vi "Retrieve_GetImage.vi"(6 "File and Directory Blacklist":string[](array[string]), 8 "error in (no error)":errorcluster, 9 "Image Metadata in":T2={"title"="", "description"="", "ID"="", "version"="", "component type"=5} {"component type" items=["standard", "hidden", "system", "unknown", "startup", "image", "essential"]}, 10 "Image Filepath":path, 11 "DevInfo":T1={"Hostname"="", "IPAddress"="", "MAC"="", "SerialNum"="", "Model"="", "Status"="", "FW"="", "OSDesc"="", "ImgTitle"="", "ImgDesc"="", "ImgVer"="", "ImgID"="", "IP Address Request Mode"=1, "SubnetMask"="", "Gateway"="", "DNSServer"=""} {"IP Address Request Mode" items=["Static"=1, "DHCP/Link-Local"=2, "Link-Local Only"=4, "DHCP Only"=8]}) -> (0 "error out":errorcluster)   [LabVIEW 2021]
uses:
  <vilib>/nisyscfg/Software 1.2.ctl
  <vilib>/nisyscfg/Component Type.ctl
  TypeDefs/DevInfo.ctl
  TypeDefs/TargetAccess.ctl
  <vilib>/nisyscfg/Create System Image (File).vi
  <vilib>/nisyscfg/Close (System).vi
  <vilib>/nisyscfg/nisyscfg.lvlib
panel:
  out "Progress":i8(slide) scale=0.0..100.0
  out "Status":string
  in  "Stop Checking for Events":bool
  # "Retrieving application image..."
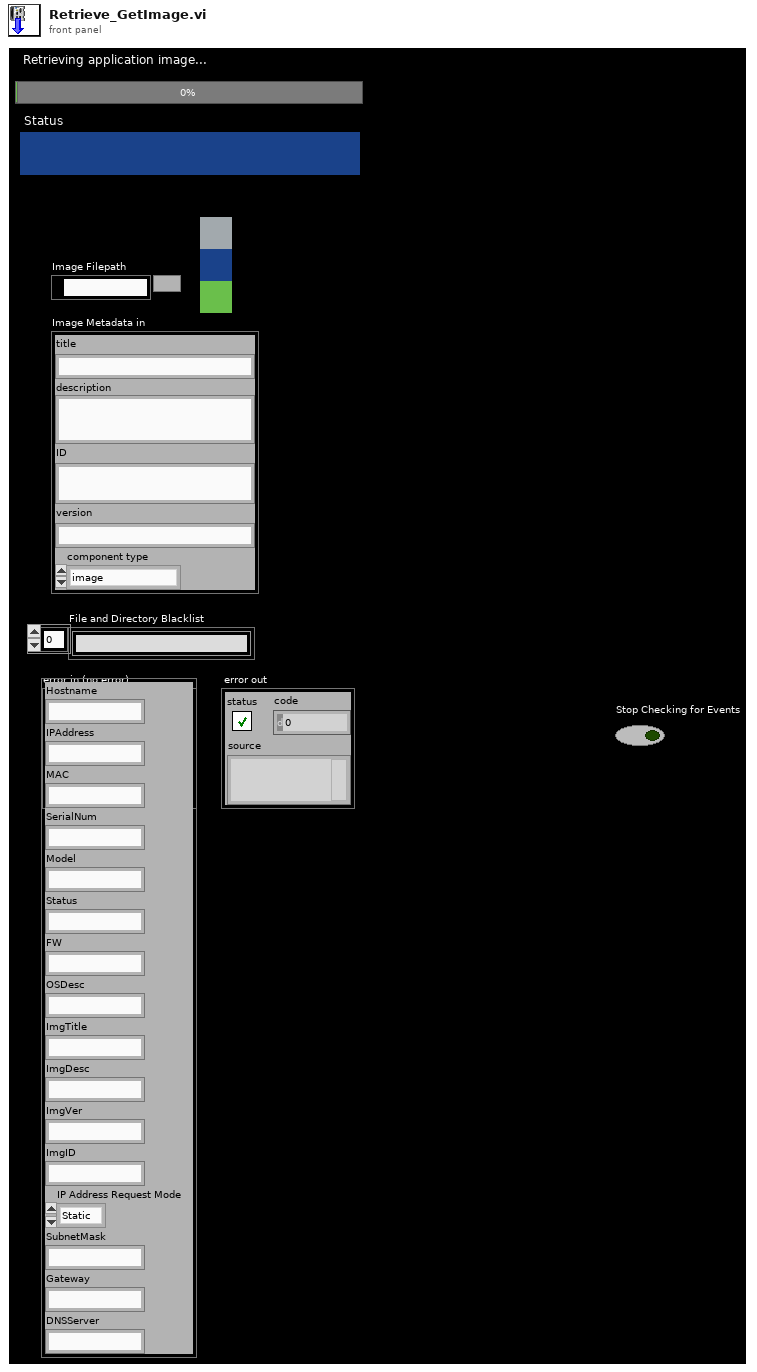
[diagram p1: front panel]
types:
  T1 = typedef "DevInfo.ctl" = cluster{"Hostname":string, "IPAddress":string, "MAC":string, "SerialNum":string, "Model":string, "Status":string, "FW":string, "OSDesc":string, "ImgTitle":string, "ImgDesc":string, "ImgVer":string, "ImgID":string, "IP Address Request Mode":i32, "SubnetMask":string, "Gateway":string, "DNSServer":string}
  T2 = typedef "nisyscfg.lvlib/Software 1.2.ctl" = cluster{"title":string, "description":string, "ID":string, "version":string, "component type":T3}
  T3 = typedef "nisyscfg.lvlib/Component Type.ctl" = u32
  T4 = typedef "TargetAccess.ctl" = enum16{"Read-Only", "Admin"}
  T5 = enum32{"state changed", "beginning restart", "getting file", "putting file", "creating directory", "deleting file", "deleting directory", "enumerating file system", "renaming file", "current component", "operation progress", "downloading file", "unpacking file", "running install script", "creating image", "validating image", "applying image", "beginning format", "completing format"}
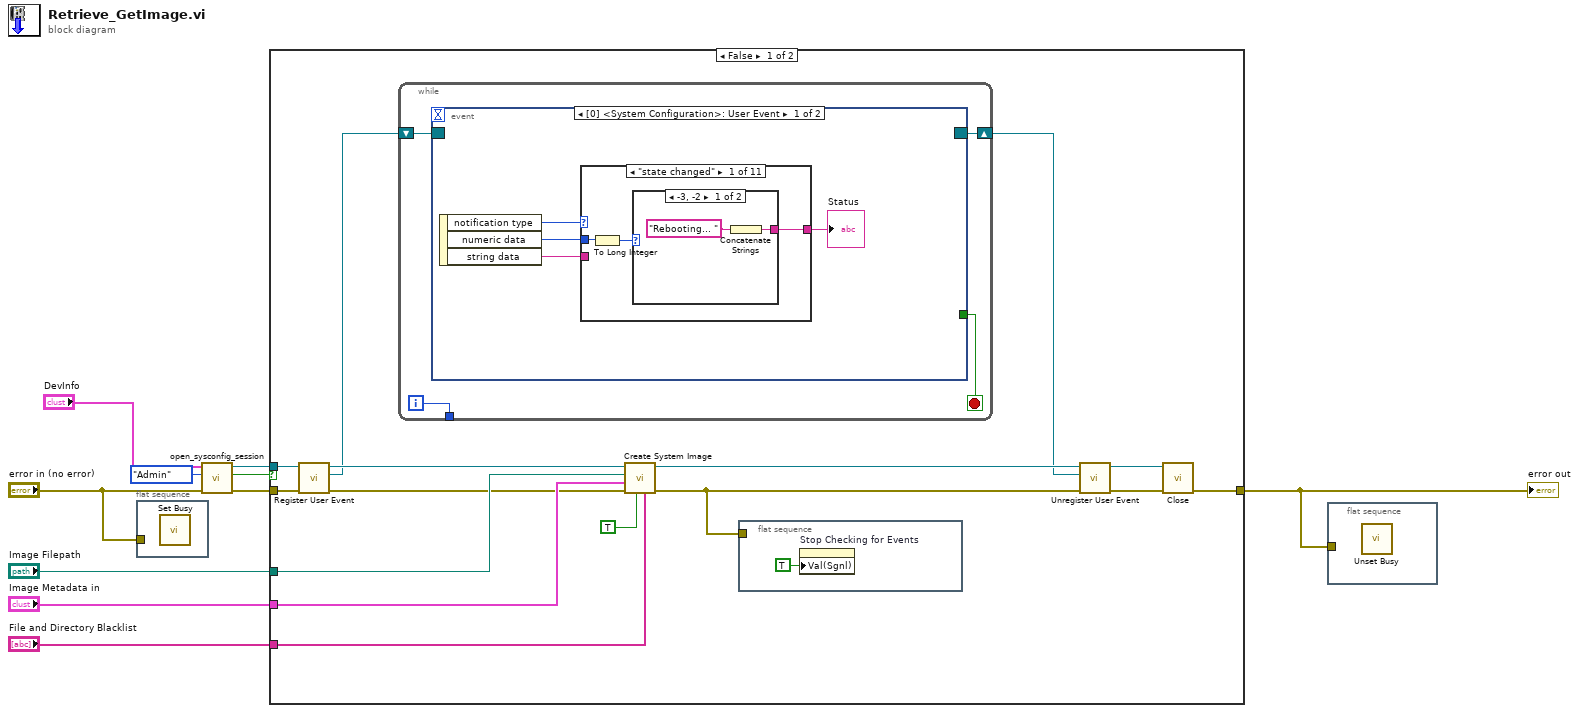
[diagram p0: block diagram]
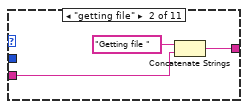
[diagram p3: hidden frame]
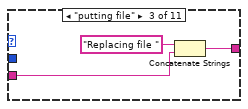
[diagram p4: hidden frame]
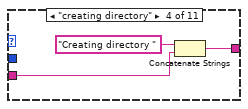
[diagram p5: hidden frame]
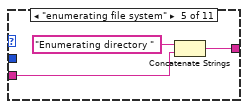
[diagram p6: hidden frame]
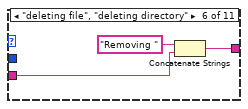
[diagram p7: hidden frame]
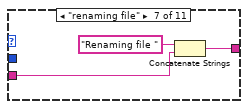
[diagram p8: hidden frame]
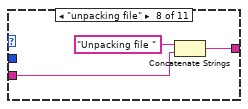
[diagram p9: hidden frame]
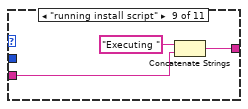
[diagram p10: hidden frame]
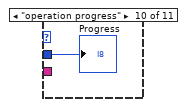
[diagram p11: hidden frame]
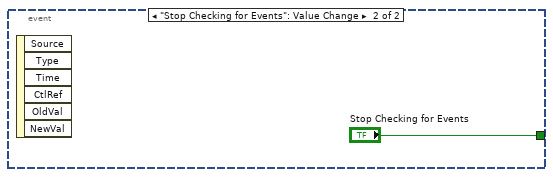
[diagram p13: hidden frame]
diagram:
  n1 = flat-sequence {
    tunnel: "error in (no error)" -> [_]
    frame #0 {
      n2 = call <vilib>:"Set Busy.vi"() -> ()  [unwired: 10 in, 2 out]
    }
  }
  n3 = call "open_sysconfig_session.vi"("error in (no error)"="error in (no error)", "Target Access"=TargetAccess."Admin", "DevInfo"="DevInfo") -> ("error out"=w7:errorcluster, "Cancelled"=w5:bool, "Session Out"=w6:refnum<k21>)  [unwired: 6 in]
  n4 = case shown="False" w5 {
    tunnel: "Image Filepath" -> [w23 _]
    tunnel: [w17 w66] -> w2
    tunnel: "File and Directory Blacklist" -> [w15 _]
    tunnel: "Image Metadata in" -> [w14 _]
    tunnel: w7 -> [w12 w66]
    tunnel: w6 -> [w11 _]
    frame False {
      n5 = call <vilib>:"Register User Event.vi"("error in (no error)"=w12, "Session in"=w11) -> ("error out"=w13:errorcluster, "Event Registration out"=w22:refnum<event-registration>, "Session out"=w24:refnum<k21>)  [unwired: 7 in]
      n6 = while {
        shift-right: [w28] -> w20
        shift-left: w22 -> [w30]
        tunnel: [w27] -> _
        i -> [w27]
        stop <- w29 stop-if-true
        n7 = event shown="[0] <System Configuration>: User Event" {
          selector: w30 -> [_ _]
          dyn-events: [_ _] -> w28
          timeout: _ -> [_ _]
          tunnel: [_ "Stop Checking for Events"] -> w29
          event User Event {
            n8 = event-data() -> ("notification type"=w34:T5, "numeric data"=w33:u32, "string data"=w32:string)  [unwired: 1 in]
            n9 = case shown="\"state changed\"" w34 {
              tunnel: [w35 w40 w43 w46 w49 w52 w55 w58 w61 _ _] -> w31
              tunnel: w32 -> [_ w41 w44 w47 w50 w53 w56 w59 w62 _ _]
              tunnel: w33 -> [w37 _ _ _ _ _ _ _ _ w64 _]
              frame "state changed" {
                n10 = To Long Integer(number=w37) -> (32bit integer=w36:i32)
                n11 = case shown="-3, -2" w36 {
                  tunnel: [w38 _] -> w35
                  frame -3, -2 {
                    n12 = Concatenate Strings("Rebooting... ") -> (w38:string)
                  }
                  frame Default {
                  }
                }
              }
              frame "getting file" {
                n13 = Concatenate Strings("Getting file " ("Status"), w41) -> (w40:string)
              }
              frame "putting file" {
                n14 = Concatenate Strings("Replacing file " ("Status"), w44) -> (w43:string)
              }
              frame "creating directory" {
                n15 = Concatenate Strings("Creating directory " ("Status"), w47) -> (w46:string)
              }
              frame "enumerating file system" {
                n16 = Concatenate Strings("Enumerating directory " ("Status"), w50) -> (w49:string)
              }
              frame "deleting file", "deleting directory" {
                n17 = Concatenate Strings("Removing " ("Status"), w53) -> (w52:string)
              }
              frame "renaming file" {
                n18 = Concatenate Strings("Renaming file " ("Status"), w56) -> (w55:string)
              }
              frame "unpacking file" {
                n19 = Concatenate Strings("Unpacking file " ("Status"), w59) -> (w58:string)
              }
              frame "running install script" {
                n20 = Concatenate Strings("Executing " ("Status"), w62) -> (w61:string)
              }
              frame "operation progress" {
                "Progress" <- w64
              }
              frame Default {
              }
            }
            "Status" <- w31
          }
          event "Stop Checking for Events": Value Change {
            n21 = event-data() -> ()  [unwired: 1 in, 6 out]
          }
        }
      }
      n22 = call-poly <vilib>:"Create System Image.vi"("File and Directory Blacklist"=w15, "Overwrite (F)"=TRUE, "error in (no error)"=w13, "Image Metadata in"=w14, "Destination File"=w23, "Session in"=w24) -> ("error out"=w18:errorcluster, "Session out"=w21:refnum<k21>)  [unwired: 3 in, 1 out]
      n23 = flat-sequence {
        tunnel: w18 -> [_]
        frame #0 {
          n24 = property on="Stop Checking for Events" class="Bool (strict)"("Val(Sgnl)"=TRUE ("Value (Signaling)")) -> ()  [unwired: 2 in, 2 out]
        }
      }
      n25 = call <vilib>:"Unregister User Event.vi"("error in (no error)"=w18, "Event Registration in"=w20, "Session in"=w21) -> ("error out"=w19:errorcluster, "Session out"=w25:refnum<k21>)  [unwired: 7 in]
      n26 = call-poly <vilib>:"Close.vi"("error in (no error)"=w19, "Session in"=w25) -> ("error out"=w17:errorcluster)  [unwired: 9 in]
    }
    frame True {
    }
  }
  "error out" <- w2
  n27 = flat-sequence {
    tunnel: w2 -> [_]
    frame #0 {
      n28 = call <vilib>:"Unset Busy.vi"() -> ()  [unwired: 11 in, 1 out]
    }
  }
